vi "Constants.vi"() -> ()   [LabVIEW 2024, in "Nominal Client Shared.lvlib"]
doc: "Use this Global VI to access the GUIDs assigned to the page resources of the Custom Device."
uses:
  Nominal Client Shared.lvlib
panel:
  in  "Tab Control":enum32{"GUIDs", "Constants", "Properties"}(tab)
  in  "Extra 3":string="e674c79a-daf8-4a81-a58e-5ae95142a496"
  in  "Extra 2":string="60bbeea1-07d5-4bd0-9c74-3dbf78c2c5e4"
  in  "Enable Streaming":string="298e9326-2f09-4be8-abaa-0ca5aecff365"
  in  "Nominal Client":string="148559e2-b901-4b9f-bf6f-5787e8eba09e"
  in  "Compiled.Settings":string="Compiled.Settings"
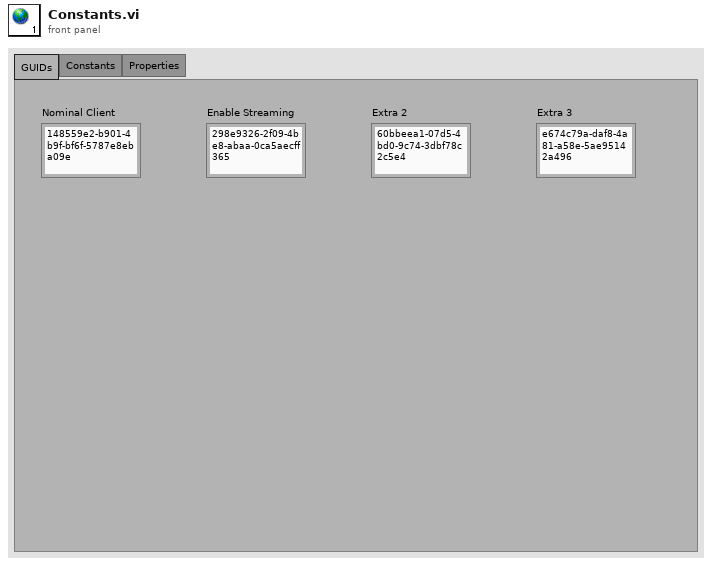
[diagram p1: front panel]
diagram:
